vi "ReadMessages.vi"(6 "Timeout(ms)":i32, 8 "error in (no error)":errorcluster, 11 "NetworkConnection in":refnum<class "NetworkConnection.lvclass">) -> (0 "error out":errorcluster, 1 "Messages":T1[](array[typedef]), 2 "StillConnected?":bool, 3 "NetworkConnection out":refnum<class "NetworkConnection.lvclass">, 4 "Timed Out?":bool)   [LabVIEW 2020, in "NetworkConnection.lvclass"]
doc: "Reads all available messages from the Remote System on the Network Connection for the desired timeout period.\n\nJKI Network Streams Connection 1.1.1.15\nJavier Ruiz - JKI\nCopyright (c) 2020, JKI\n\nThis library is provided \"AS IS\" ,WITHOUT WARRANTIES OR CONDITIONS OF ANY KIND, either express or implied."
uses:
  NetworkConnection.lvclass
  NetworkCommand--Cluster.ctl
  NetworkConnection.lvclass/NetworkConnection.ctl
panel:
  # "Copyright © 2020 JKI All rights reserved.\n\nAuthor: Javier Ruiz <javier.ruiz@jki.net>\n\nThis library is provided \"AS IS\" ,WITHOUT WARRANTIES OR \nCONDITIONS OF ANY KIND, either expressed or implied.\n\nJKI -- jki.net"
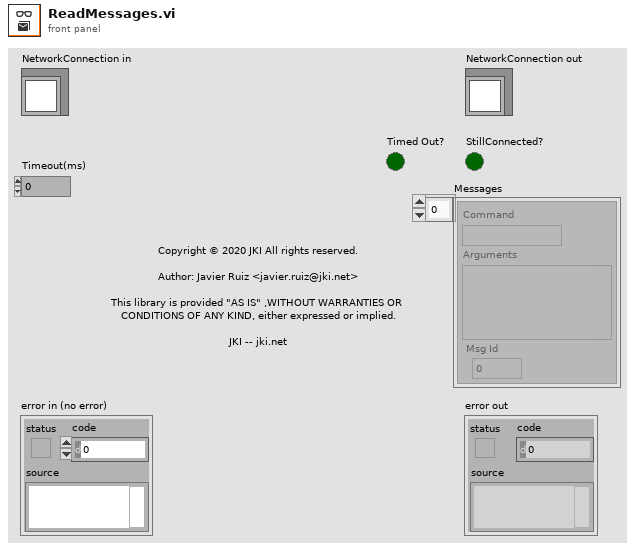
[diagram p1: front panel]
types:
  T1 = typedef "NetworkConnection.lvclass/NetworkCommand--Cluster.ctl" = cluster{"Command":string, "Arguments":variant, " Msg Id":i32}
  T2 = typedef "NetworkConnection.lvclass/NetworkMessage--Cluster.ctl" = cluster{"NetworkCommand":T1, "Wait for Ack?":bool, "Ack Id":i32}
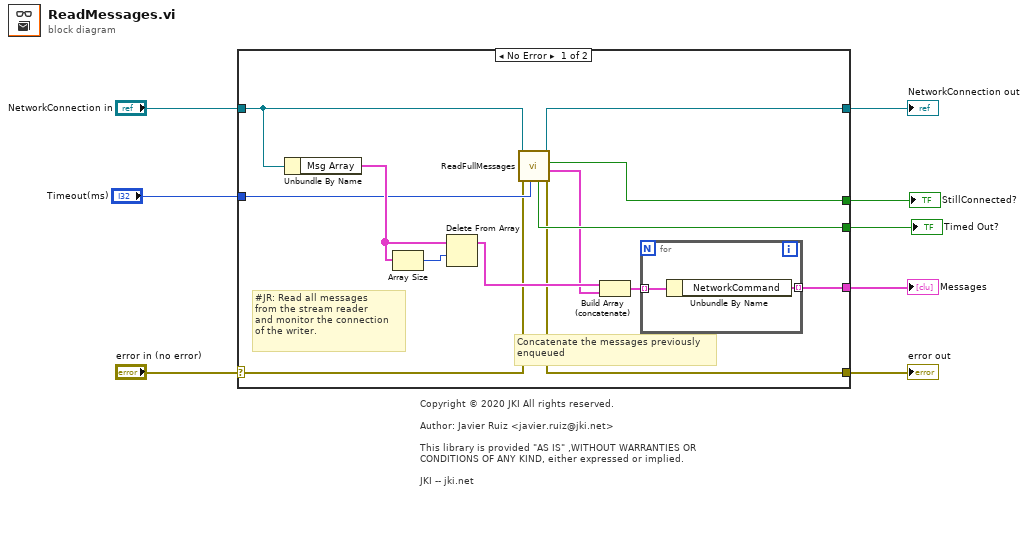
[diagram p0: block diagram]
diagram:
  # "Copyright © 2020 JKI All rights reserved.\n\nAuthor: Javier Ruiz <javier.ruiz@jki.net>\n\nThis library is provided \"AS IS\" ,WITHOUT WARRANTIES OR \nCONDITIONS OF ANY KIND, either expressed or implied.\n\nJKI -- jki.net"
  n1 = case shown="No Error" "error in (no error)" {
    selector: "error in (no error)" -> [w10 w25]
    tunnel: [w9 w25] -> w7
    tunnel: [w15 w24] -> w5
    tunnel: "NetworkConnection in" -> [w16 w24]
    tunnel: "Timeout(ms)" -> [w14 _]
    tunnel: [w17 _] -> w3
    tunnel: [w11 _] -> w2
    tunnel: [w13 _] -> w1
    frame No Error {
      # "Concatenate the messages previously\nenqueued"
      # "#JR: Read all messages\nfrom the stream reader\nand monitor the connection\nof the writer."
      n2 = Unbundle By Name(w16) -> ("Msg Array"=w20:T2[])
      n3 = Array Size(array=w20) -> (size(s)=w21:i32)
      n4 = Delete From Array(array=w20, length=w21) -> (array with subset deleted=w19:T2[])  [unwired: 1 in, 1 out]
      n5 = call "ReadFullMessages.vi"("Timeout(ms)"=w14, "error in (no error)"=w10, "NetworkConnection in"=w16) -> ("error out"=w9:errorcluster, "Messages"=w12:T2[], "StillConnected?"=w11:bool, "NetworkConnection out"=w15:refnum<class "NetworkConnection.lvclass">, "Timed Out?"=w13:bool)  [unwired: 4 in]
      n6 = Build Array (concatenate)(w19, w12) -> (w18:T2[])
      n7 = for {
        tunnel: w18 -> [w23] mode=indexing
        tunnel: [w22] -> w17 mode=indexing
        n8 = Unbundle By Name(w23) -> ("NetworkCommand"=w22:T1)
      }
    }
    frame Error {
    }
  }
  "error out" <- w7
  "NetworkConnection out" <- w5
  "StillConnected?" <- w2
  "Messages" <- w3
  "Timed Out?" <- w1
